vi "Rollover handler (Core).vi"(9 "Target delay":u32, 11 "Tick Count Register in":u32) -> (0 "Target delay reached":bool, 1 "Raw count":u32, 2 "Elapsed ticks count":u32, 3 "Tick Count Register out":u32)   [LabVIEW 2020]
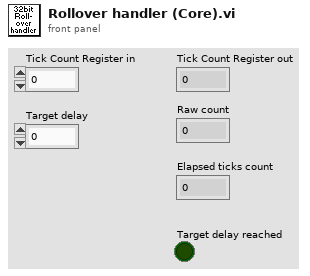
[diagram p1: front panel]
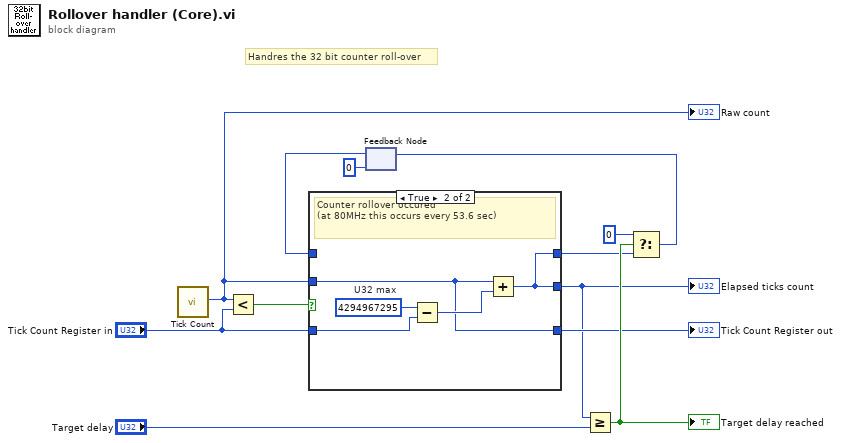
[diagram p0: block diagram]
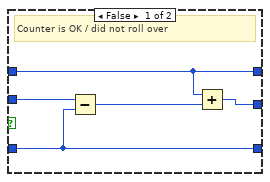
[diagram p2: hidden frame]
diagram:
  # "Handres the 32 bit counter roll-over"
  n1 = call "Tick Count"() -> ("Tick Count(Ticks)"=w8:u32)
  "Raw count" <- w8
  n2 = Less?(x=w8, y="Tick Count Register in") -> (x < y?=w2:bool)
  n3 = feedback #1(u32 0) -> (w3:u32)
  n4 = case shown="True" w2 {
    tunnel: w8 -> [w17 w19]
    tunnel: "Tick Count Register in" -> [w16 w21]
    tunnel: [w14 w18] -> w9
    tunnel: [w16 w19] -> w10
    tunnel: [w13 w18] -> w6
    tunnel: w3 -> [w13 _]
    frame False {
      # "Counter is OK / did not roll over"
      n5 = Subtract(x=w17, y=w16) -> (x-y=w15:u32)
      n6 = Add(x=w13, y=w15) -> (x+y=w14:u32)
    }
    frame True {
      w22 = u32 4294967295  # U32 max
      # "Counter rollover occured\n(at 80MHz this occurs every 53.6 sec)"
      n7 = Subtract(x=w22, y=w21) -> (x-y=w20:u32)
      n8 = Add(x=w19, y=w20) -> (x+y=w18:u32)
    }
  }
  "Tick Count Register out" <- w10
  "Elapsed ticks count" <- w9
  n9 = Greater Or Equal?(x=w9, y="Target delay") -> (x >= y?=w11:bool)
  "Target delay reached" <- w11
  n10 = Select(t=u32 0, s=w11, f=w6) -> (s? t:f=w5:u32)
  n11 = feedback-in #1(w5) -> ()
